vi "Constant_Extension_FileName.vi"() -> (0 "File Name String":string="fraw")   [LabVIEW 2018]
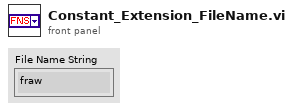
[diagram p1: front panel]
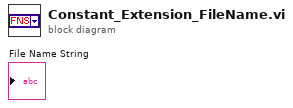
[diagram p0: block diagram]
diagram:
